vi "LoadInlineData.vi"(8 "error in (no error)":errorcluster, 10 "VI Refnum":refnum<vi>) -> (0 "error out":errorcluster, 2 "Inline Data":string[](array[string]))   [LabVIEW 2019]
uses:
  <vilib>/JDP Science/JSONtext/JSONtext.lvlib
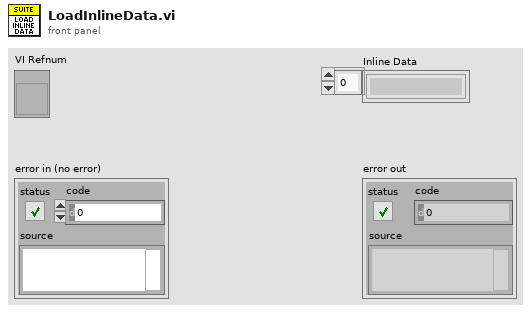
[diagram p1: front panel]
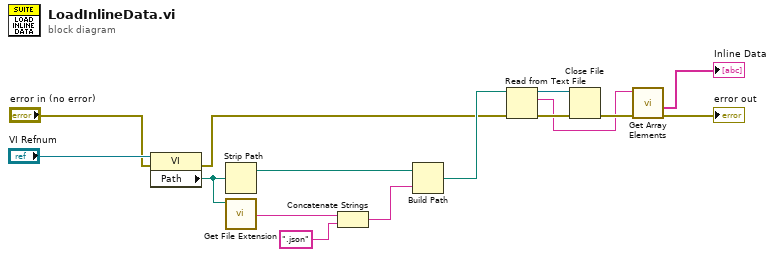
[diagram p0: block diagram]
diagram:
  n1 = property class="VI"(reference="VI Refnum", error in="error in (no error)") -> (error out=w1:errorcluster, "Path"=w2:path)  [unwired: 1 out]
  n2 = Strip Path(path=w2) -> (stripped path=w9:path)  [unwired: 1 out]
  n3 = call <vilib>:"Get File Extension.vi"("file"=w2) -> ("filename without extension"=w11:string)  [unwired: 6 in, 4 out]
  n4 = Concatenate Strings(w11, ".json" ("string")) -> (w8:string)
  n5 = Build Path(base path=w9, name or relative path=w8) -> (appended path=w7:path)
  n6 = Read from Text File(file (use dialog)=w7, error in=w1) -> (refnum out=w4:refnum<file>, text=w3:string, error out=w6:errorcluster)  [unwired: 2 in, 1 out]
  n7 = Close File(refnum=w4, error in=w6) -> (error out=w5:errorcluster)  [unwired: 1 out]
  n8 = call <vilib>:"Get Array Elements.vi"("error in (no error)"=w5, "JSON"=w3) -> ("error out"=→"error out":errorcluster, "<JSON>"=→"Inline Data":string[])  [unwired: 7 in, 1 out]
